vi "Ex. 1. Build Your First Application.vi"() -> ()   [LabVIEW 2024]
uses:
  <vilib>/measure/NI_MABase.lvlib
panel:
  in  "Stop":bool
  out "Time Domain Signal":waveform(dbl)(graph)
  in  "Frequency":dbl(knob) scale=0.0..50.0
  # "Signal Generation Demo"
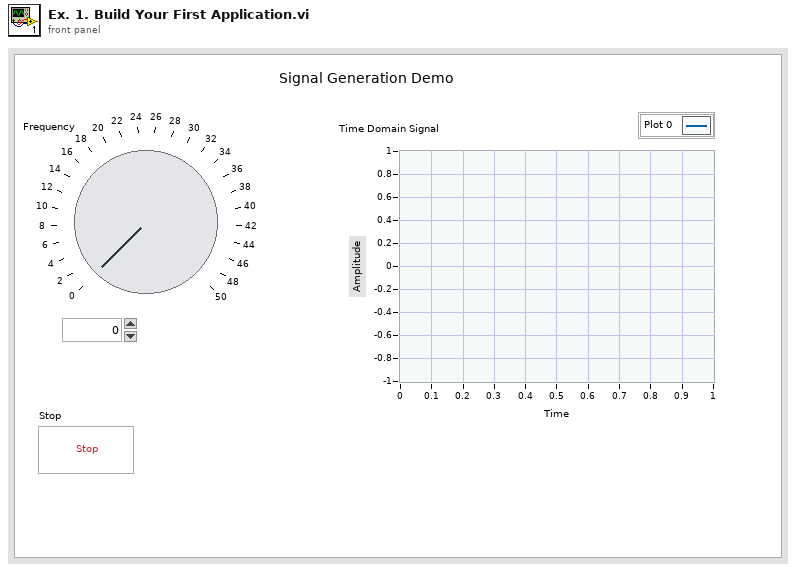
[diagram p1: front panel]
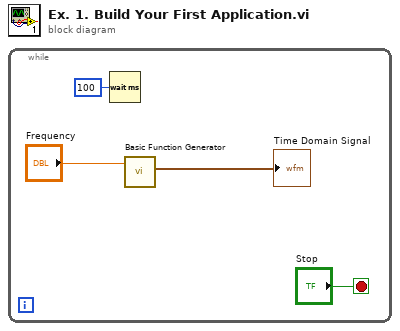
[diagram p0: block diagram]
diagram:
  n1 = while {
    stop <- "Stop" stop-if-true
    n2 = Wait (ms)(milliseconds to wait=u32 100) -> ()  [unwired: 1 out]
    n3 = call <vilib>:"Basic Function Generator.vi"("frequency"="Frequency") -> ("signal out"=→"Time Domain Signal":waveform(dbl))  [unwired: 8 in, 2 out]
  }
